vi "configure.vi"(8 "error in (no error)":errorcluster, 9 "write enable":bool=TRUE, 11 "MB_TCP in":refnum<class "MB_TCP.lvclass">) -> (0 "error out":errorcluster, 3 "MB_TCP out":refnum<class "MB_TCP.lvclass">)   [LabVIEW 2021, in "MB_TCP.lvclass"]
uses:
  MB_TCP.lvclass
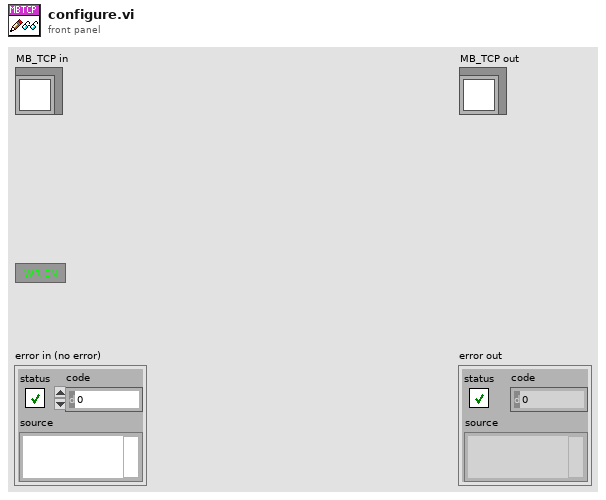
[diagram p1: front panel]
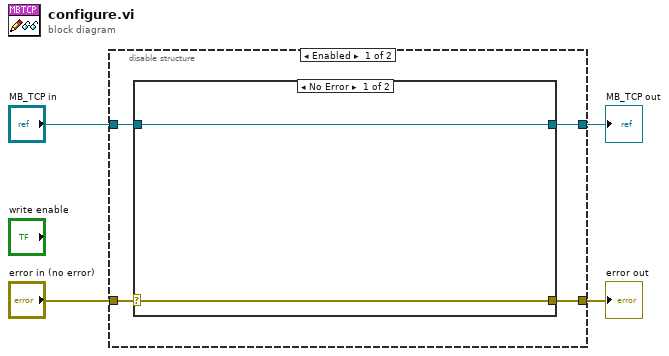
[diagram p0: block diagram]
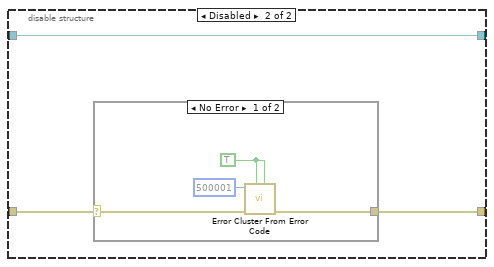
[diagram p3: hidden frame]
diagram:
  n1 = disable-structure shown="Enabled" {
    disable-tunnel: "error in (no error)" -> [w8 w13]
    disable-tunnel: [w7 w14] -> w3
    disable-tunnel: "MB_TCP in" -> [w6 w15]
    disable-tunnel: [w5 w15] -> w1
    frame Enabled {
      n2 = case shown="No Error" w8 {
        selector: w8 -> [w9 w12]
        tunnel: [w9 w12] -> w7
        tunnel: [w10 w11] -> w5
        tunnel: w6 -> [w10 w11]
        frame No Error {
        }
        frame Error {
        }
      }
    }
    frame Disabled {
      n3 = case shown="No Error" w13 {
        selector: w13 -> [w16 w20]
        tunnel: [w17 w20] -> w14
        frame No Error {
          w18 = TRUE ("show call chain? (False)")
          n4 = call <vilib>:"Error Cluster From Error Code.vi"("is warning? (False)"=w18, "show call chain? (False)"=w18, "error in (no error)"=w16, "error code (0)"=500001) -> ("error out"=w17:errorcluster)  [unwired: 5 in]
        }
        frame Error {
        }
      }
    }
  }
  "error out" <- w3
  "MB_TCP out" <- w1
